vi "Metadata - database.vi"(8 "error in (no error)":errorcluster, 10 "Database in":string, 11 "mysql in":refnum<class "mysql.lvclass">) -> (0 "error out":errorcluster, 2 "Database metadata":string[][](array[string]), 3 "mysql out":refnum<class "mysql.lvclass">)   [LabVIEW 2020, in "mysql.lvlib" / "mysql.lvclass"]
uses:
  mysql.lvclass
  1b66d04b-d4ed-4884-b7e3-1172a05fde65.vi
  <vilib>/Utility/error.llb/Error Cluster From Error Code.vi
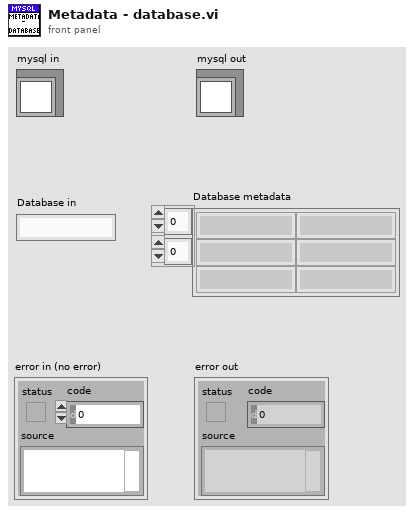
[diagram p1: front panel]
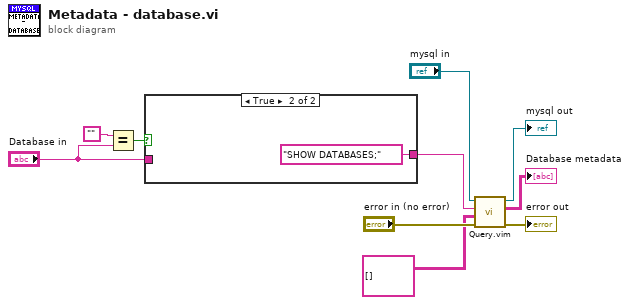
[diagram p0: block diagram]
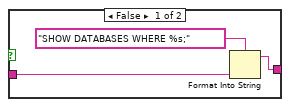
[diagram p2: hidden frame]
diagram:
  n1 = Equal?(x="", y="Database in") -> (x = y?=w7:bool)
  n2 = case shown="True" w7 {
    tunnel: [w12 "SHOW DATABASES;" ("format string")] -> w9
    tunnel: "Database in" -> [w11 _]
    frame False {
      n3 = Format Into String(format string="SHOW DATABASES WHERE %s;", w11) -> (resulting string=w12:string)  [unwired: 2 in, 1 out]
    }
    frame True {
    }
  }
  n4 = call "Query.vim"("error in (no error)"="error in (no error)", "Type and Default"=string[][] [] ("Database metadata 2"), "Query string"=w9, "IDatabase in"="mysql in") -> ("error out"=→"error out":errorcluster, "Result"=→"Database metadata":string[][], "IDatabase out"=→"mysql out":refnum<class "mysql.lvclass">)  [unwired: 5 in]
